vi "FTW-Container-Array-Elements.vi"(0 "FTW-Container In":refnum<class "FTW-Container.lvclass">, 11 "error in":errorcluster) -> (4 "FTW-Container Out":refnum<class "FTW-Container.lvclass">, 6 "Array Elements":refnum<class "FTW-Container.lvclass">[](array[class]), 15 "error out":errorcluster)   [LabVIEW 2015, in "FTW-Container.lvclass"]
uses:
  FTW-Container.lvclass
  FTW-Container.lvclass/FTW-Container.ctl
  <vilib>/Utility/Data Type/NI_Data Type.lvlib
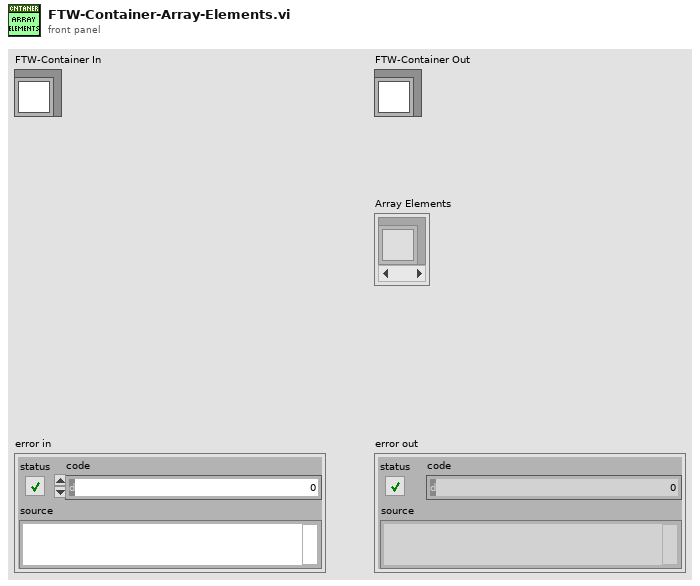
[diagram p1: front panel]
types:
  T1 = typedef "NI_Data Type.lvlib/Data Type.ctl" = enum8{"Invalid Type", "Void", "I8", "I16", "I32", "I64", "U8", "U16", "U32", "U64", "Single Float", "Double Float", "Extended Float", "Single Complex", "Double Complex", "Extended Complex", "Enum U8", "Enum U16", "Enum U32", "Enum U64", "Single Float With Unit", "Double Float With Unit", "Extended Float With Unit", "Single Complex with Unit", "Double Complex with Unit", "Extended Complex with Unit", "Boolean", "String", "Path", "Picture", "Tag", "Array", "Cluster", "Variant", "LV Variant", "Waveform", "Timestamp", "Digital Waveform", "Digital Data", "ExpressData", "Refnum", "External Data", "VI", "Poly VI", "LabVIEW Class Instance", "Fixed Point"}
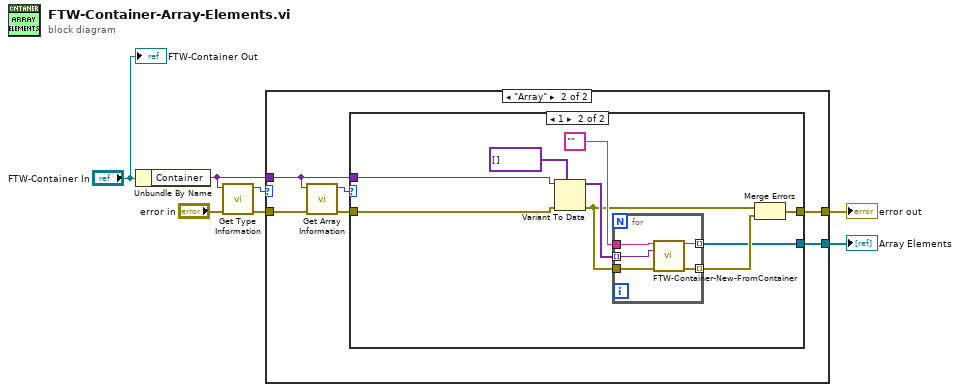
[diagram p0: block diagram]
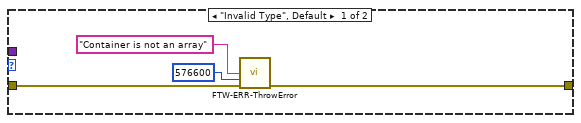
[diagram p2: hidden frame]
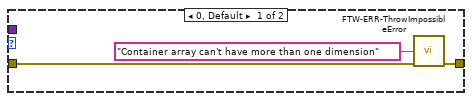
[diagram p3: hidden frame]
diagram:
  n1 = Unbundle By Name("FTW-Container In") -> ("Container"=w2:variant)
  n2 = call <vilib>:"Get Type Information.vi"("error in (no error)"="error in", "Variant"=w2) -> ("error out"=w5:errorcluster, "Type"=w1:T1)  [unwired: 5 in, 3 out]
  n3 = case shown="\"Array\"" w1 {
    tunnel: w5 -> [w11 w15]
    tunnel: [w10 w14] -> w4
    tunnel: [_ w13] -> w3
    tunnel: w2 -> [_ w12]
    frame "Invalid Type", Default {
      n4 = call "FTW-ERR-ThrowError.vi"("Error Message"="Container is not an array", "Error Code"=576600, "error in"=w11) -> ("error out"=w10:errorcluster)  [unwired: 12 in]
    }
    frame "Array" {
      n5 = call <vilib>:"Get Array Information.vi"("error in (no error)"=w15, "Variant"=w12) -> ("error out"=w17:errorcluster, "Number of Dimensions"=w16:i32)  [unwired: 6 in, 2 out]
      n6 = case shown="1" w16 {
        tunnel: w17 -> [w20 w28]
        tunnel: w12 -> [_ w27]
        tunnel: [w19 w23] -> w14
        tunnel: [_ w21] -> w13
        frame 0, Default {
          n7 = call "FTW-ERR-ThrowImpossibleError.vi"("Reason this error should never happen"="Container array can't have more than one dimension", "error in"=w20) -> ("error out"=w19:errorcluster)  [unwired: 13 in]
        }
        frame 1 {
          n8 = Variant To Data(error in=w28, type=variant[] [], Variant=w27) -> (data=w24:variant[], error out=w22:errorcluster)
          n9 = for {
            tunnel: "" ("empty string") -> [w32]
            tunnel: w24 -> [w31] mode=indexing
            tunnel: w22 -> [w34]
            tunnel: [w33] -> w26 mode=indexing
            tunnel: [w30] -> w21 mode=indexing
            n10 = call "FTW-Container-New-FromContainer.vi"("Name"=w32, "Container"=w31, "error in"=w34) -> ("FTW-Container"=w30:refnum<class "FTW-Container.lvclass">, "error out"=w33:errorcluster)  [unwired: 11 in]
          }
          n11 = Merge Errors(w22, w26) -> (w23:errorcluster)
        }
      }
    }
  }
  "error out" <- w4
  "Array Elements" <- w3
  "FTW-Container Out" <- "FTW-Container In"
